vi "display_michelle_PKT_visjitter_stopadded_ContrastTitration.vi"() -> ()   [LabVIEW 2019]
uses:
  <vilib>/Analysis/Matrix/Datatypes/RealMatrix.ctl
  <vilib>/Utility/file.llb/Write Delimited Spreadsheet (DBL).vi
  <vilib>/Analysis/Matrix/NI_Matrix.lvlib
panel:
  out "lambda":dbl
  out "maxITI":dbl
  out "minITI":dbl
  out "goEXP":dbl
  out "Array temp3":T1
  out "OTDisp":dbl
  out "Performance":dbl
  out "CurrentContrast":dbl
  out "OTRew":dbl
  out "TrialGroup":dbl format="%#_13g"
  out "DisplayCount":dbl
  out "TimeOutCounter":i32
  out "ElapsedTime_M":dbl
  out "IMG_Contrast":dbl
  out "CurrentTrial":u32=1
  out "Jitter":dbl
  out "BaseITI":dbl
  out "VisStimDuration":dbl
  in  "Stop":bool
  out "Num trials":u32=204
  out "ISI Time":dbl
  out "Stim TS":dbl
  out "Output":dbl[][](array[numeric])
  out "Output frame":T1
  out "Array temp1":T1
  out "Elapsed Time":dbl
  out "Display":bool=TRUE
  out "Trial":u32=1
  out "reward":dbl[](array[numeric])
  out "stim_id":dbl[](array[numeric])
  out "stim_loaded":dbl
  out "Timings":dbl[](array[numeric])
  out "Stimuli Loaded?":bool
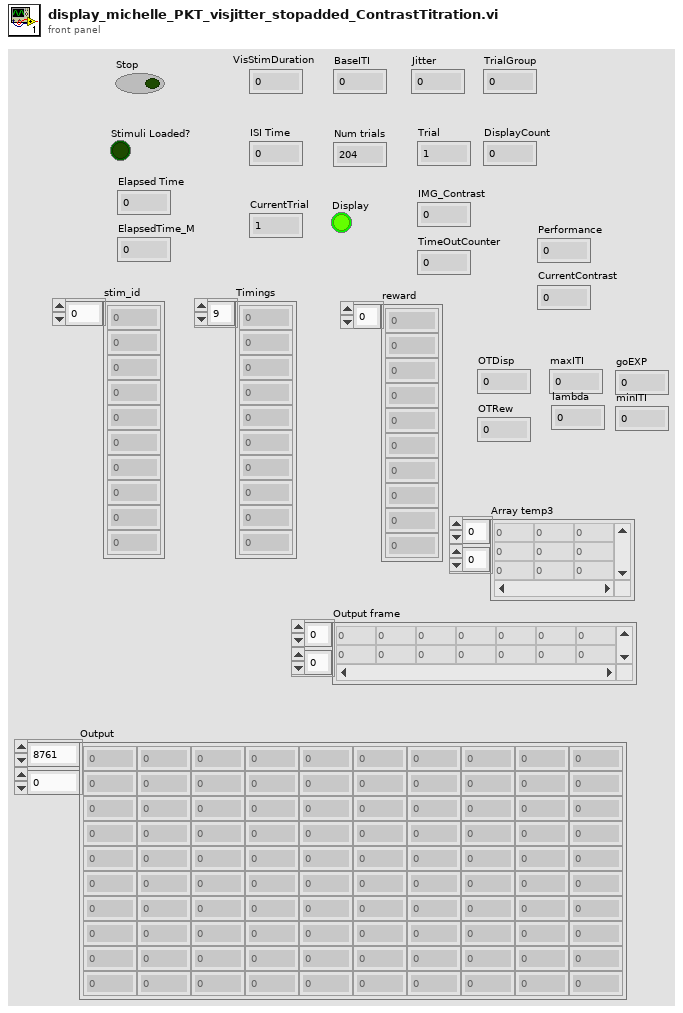
[diagram p1: front panel]
types:
  T1 = typedef "NI_Matrix.lvlib/RealMatrix.ctl" = dbl[][]
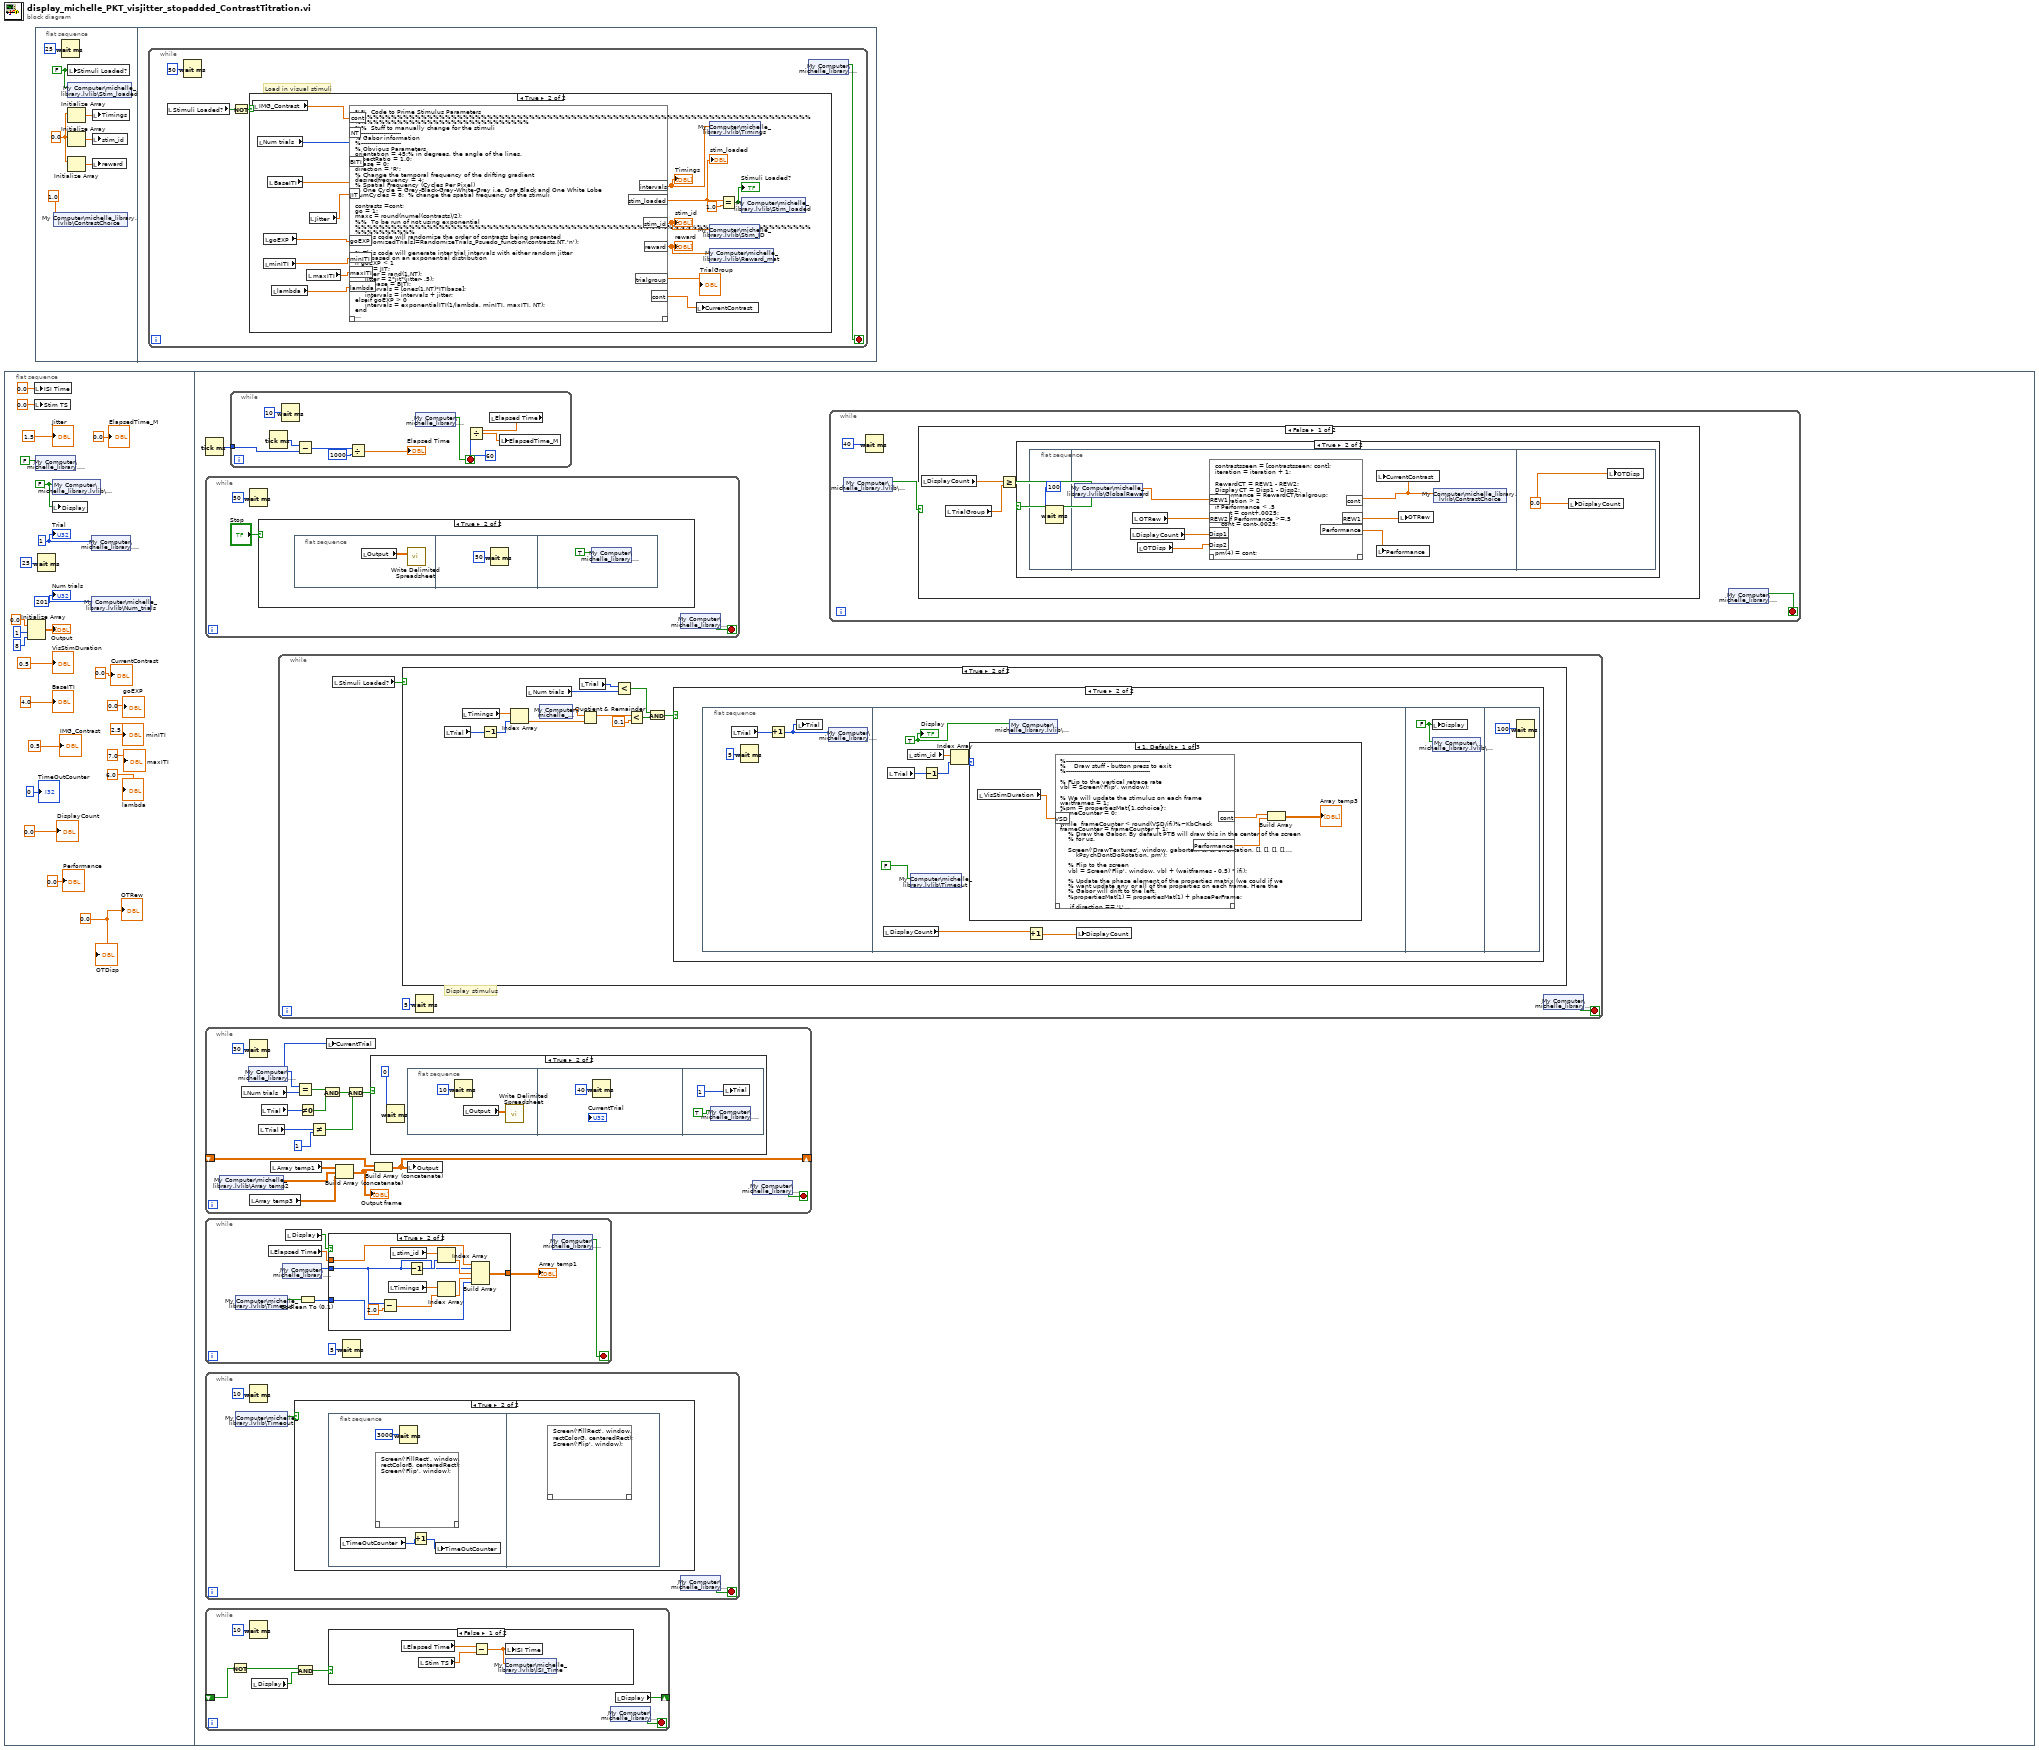
[diagram p0: block diagram]
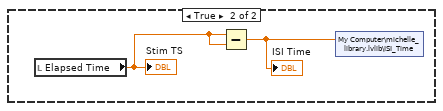
[diagram p7: hidden frame]
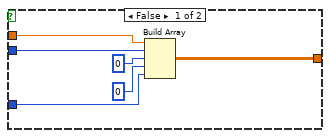
[diagram p8: hidden frame]
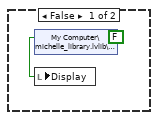
[diagram p11: hidden frame]
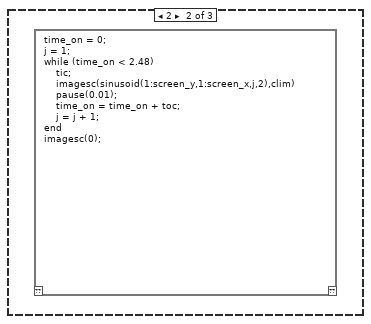
[diagram p12: hidden frame]
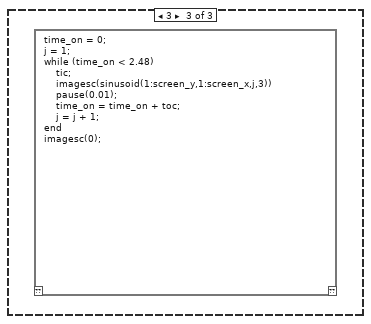
[diagram p13: hidden frame]
diagram:
  n1 = flat-sequence {
    frame #0 {
      w7 = 0.0
      w17 = u32 201
      w23 = FALSE ("Display")
      w25 = u32 1 ("Trial")
      n2 = Initialize Array(0.0 ("element"), 1 ("dimension size"), 8 ("dimension size")) -> (→"Output":dbl[][])
      n3 = local write "ISI Time"(0.0 ("ISI Time")) -> ()
      n4 = local write "Stim TS"(0.0 ("Stim TS")) -> ()
      n5 = shared-variable "My Computer\\michelle_library.lvlib\\Stop"(FALSE ("Stop")) -> ()  [unwired: 1 in, 1 out]
      n6 = Wait (ms)(milliseconds to wait=u32 25) -> ()  [unwired: 1 out]
      n7 = shared-variable "My Computer\\michelle_library.lvlib\\Display"(w23) -> ()  [unwired: 1 in, 1 out]
      n8 = local write "Display"(w23) -> ()
      n9 = shared-variable "My Computer\\michelle_library.lvlib\\Trial"(w25) -> ()  [unwired: 1 in, 1 out]
      n10 = shared-variable "My Computer\\michelle_library.lvlib\\Num_trials"(w17) -> ()  [unwired: 1 in, 1 out]
      "Trial" <- w25
      "Num trials" <- w17
      "VisStimDuration" <- 0.5
      "BaseITI" <- 4.0
      "Jitter" <- 1.5
      "IMG_Contrast" <- 0.5
      "ElapsedTime_M" <- 0.0
      "TimeOutCounter" <- 0
      "DisplayCount" <- 0.0
      "OTRew" <- w7
      "CurrentContrast" <- 0.0
      "Performance" <- 0.0
      "OTDisp" <- w7
      "goEXP" <- 0.0
      "minITI" <- 2.5
      "maxITI" <- 7.0
      "lambda" <- 6.0
    }
    frame #1 {
      n11 = Tick Count (ms)() -> (millisecond timer value=w26:u32)
      n12 = while {
        stop <- w44 stop-if-true
        n13 = Wait (ms)(milliseconds to wait=50) -> ()  [unwired: 1 out]
        n14 = case shown="True" "Stop" {
          frame False {
          }
          frame True {
            n15 = flat-sequence {
              frame #0 {
                n16 = local read "Output"() -> (w45:dbl[][])
                n17 = call-poly <vilib>:"Write Delimited Spreadsheet.vi"("2D data"=w45) -> ()  [unwired: 13 in, 2 out]
              }
              frame #1 {
                n18 = Wait (ms)(milliseconds to wait=50) -> ()  [unwired: 1 out]
              }
              frame #2 {
                n19 = shared-variable "My Computer\\michelle_library.lvlib\\Stop"(TRUE) -> ()  [unwired: 1 in, 1 out]
              }
            }
          }
        }
        n20 = shared-variable "My Computer\\michelle_library.lvlib\\Stop"() -> (w44:bool)  [unwired: 1 in, 1 out]
      }
      n21 = while {
        shift-right: [w115] -> _
        shift-left: _ -> [w116]
        stop <- w118 stop-if-true
        n22 = shared-variable "My Computer\\michelle_library.lvlib\\Array temp2"() -> (w113:dbl[][])  [unwired: 1 in, 1 out]
        n23 = local read "Num trials"() -> (w111:u32)
        n24 = shared-variable "My Computer\\michelle_library.lvlib\\Trial"() -> (w102:u32)  [unwired: 1 in, 1 out]
        n25 = Wait (ms)(milliseconds to wait=u32 30) -> ()  [unwired: 1 out]
        n26 = local read "Array temp3"() -> (w101:T1)
        n27 = local read "Trial"() -> (w108:u32)
        n28 = local read "Trial"() -> (w109:u32)
        n29 = local read "Array temp1"() -> (w114:T1)
        n30 = Equal?(x=w102, y=w111) -> (x = y?=w110:bool)
        n31 = Not Equal To 0?(x=w109) -> (x != 0?=w105:bool)
        n32 = Not Equal?(x=w108, y=1) -> (x != y?=w107:bool)
        n33 = And(x=w110, y=w105) -> (x .and. y?=w103:bool)
        n34 = local write "CurrentTrial"(w102) -> ()
        n35 = Build Array (concatenate)(w114, w113, w101) -> (w112:T1)
        "Output frame" <- w112
        n36 = And(x=w103, y=w107) -> (x .and. y?=w104:bool)
        n37 = case shown="True" w104 {
          frame False {
          }
          frame True {
            n38 = Wait (ms)(milliseconds to wait=0) -> ()  [unwired: 1 out]
            n39 = flat-sequence {
              frame #0 {
                n40 = Wait (ms)(milliseconds to wait=u32 10) -> ()  [unwired: 1 out]
                n41 = local read "Output"() -> (w121:dbl[][])
                n42 = call-poly <vilib>:"Write Delimited Spreadsheet.vi"("2D data"=w121) -> ()  [unwired: 13 in, 2 out]
              }
              frame #1 {
                n43 = Wait (ms)(milliseconds to wait=u32 40) -> ()  [unwired: 1 out]
              }
              frame #2 {
                n44 = shared-variable "My Computer\\michelle_library.lvlib\\Stop"(TRUE) -> ()  [unwired: 1 in, 1 out]
                n45 = local write "Trial"(1) -> ()
              }
            }
          }
        }
        n46 = Build Array (concatenate) ("Build Matrix")(w116, w112) -> (w115:T1)
        n47 = local write "Output"(w115) -> ()
        n48 = shared-variable "My Computer\\michelle_library.lvlib\\Stop"() -> (w118:bool)  [unwired: 1 in, 1 out]
      }
      n49 = while {
        stop <- w68 stop-if-true
        n50 = shared-variable "My Computer\\michelle_library.lvlib\\Timeout"() -> (w66:bool)  [unwired: 1 in, 1 out]
        n51 = local read "Elapsed Time"() -> (w72:dbl)
        n52 = shared-variable "My Computer\\michelle_library.lvlib\\Trial"() -> (w70:u32)  [unwired: 1 in, 1 out]
        n53 = local read "Display"() -> (w69:bool)
        n54 = Boolean To (0,1)(Boolean=w66) -> (0, 1=w67:i16)
        n55 = case shown="True" w69 {
          tunnel: w70 -> [w78 w81]
          tunnel: w72 -> [w79 w88]
          tunnel: [w77 w89] -> w71
          tunnel: w67 -> [w74 w83]
          frame False {
            n56 = Build Array(w79, w78, u32 0 ("milliseconds to wait"), 0, w74) -> (w77:T1)
          }
          frame True {
            n57 = Subtract(x=w81, y=2.0) -> (x-y=w80:dbl)
            n58 = local read "Timings"() -> (w86:dbl[])
            n59 = local read "stim_id"() -> (w90:dbl[])
            n60 = Decrement(x=w81) -> (x-1=w85:u32)
            n61 = Index Array(array=w90, index=w85) -> (element=w87:dbl)
            n62 = Index Array(array=w86, index=w80) -> (element=w84:dbl)
            n63 = Build Array(w88, w81, w87, w84, w83) -> (w89:T1)
          }
        }
        "Array temp1" <- w71
        n64 = Wait (ms)(milliseconds to wait=u32 5) -> ()  [unwired: 1 out]
        n65 = shared-variable "My Computer\\michelle_library.lvlib\\Stop"() -> (w68:bool)  [unwired: 1 in, 1 out]
      }
      n66 = while {
        stop <- w50 stop-if-true
        n67 = shared-variable "My Computer\\michelle_library.lvlib\\Timeout"() -> (w48:bool)  [unwired: 1 in, 1 out]
        n68 = Wait (ms)(milliseconds to wait=u32 10) -> ()  [unwired: 1 out]
        n69 = case shown="True" w48 {
          frame False {
          }
          frame True {
            n70 = flat-sequence {
              frame #0 {
                n71 = local read "TimeOutCounter"() -> (w52:i32)
                n72 = script code="Screen('FillRect', window, rectColorB, centeredRect);\nScreen('Flip', window);"() -> ()  [unwired: 1 in, 1 out]
                n73 = Wait (ms)(milliseconds to wait=u32 3000) -> ()  [unwired: 1 out]
                n74 = Increment(x=w52) -> (x+1=w51:i32)
                n75 = local write "TimeOutCounter"(w51) -> ()
              }
              frame #1 {
                n76 = script code="Screen('FillRect', window, rectColorG, centeredRect);\nScreen('Flip', window);"() -> ()  [unwired: 1 in, 1 out]
              }
            }
          }
        }
        n77 = shared-variable "My Computer\\michelle_library.lvlib\\Stop"() -> (w50:bool)  [unwired: 1 in, 1 out]
      }
      n78 = while {
        shift-right: [w58] -> _
        shift-left: _ -> [w57]
        stop <- w60 stop-if-true
        n79 = Not(x=w57) -> (.not. x?=w56:bool)
        n80 = Wait (ms)(milliseconds to wait=u32 10) -> ()  [unwired: 1 out]
        n81 = local read "Display"() -> (w55:bool)
        n82 = And(x=w56, y=w55) -> (x .and. y?=w54:bool)
        n83 = case shown="False" w54 {
          frame False {
            n84 = local read "Elapsed Time"() -> (w61:dbl)
            n85 = local read "Stim TS"() -> (w63:dbl)
            n86 = Subtract(x=w61, y=w63) -> (x-y=w62:dbl)
            n87 = local write "ISI Time"(w62) -> ()
            n88 = shared-variable "My Computer\\michelle_library.lvlib\\ISI_Time"(w62) -> ()  [unwired: 1 in, 1 out]
          }
          frame True {
            n89 = local read "Elapsed Time"() -> (w64:dbl)
            "Stim TS" <- w64
            n90 = Subtract(x=w64, y=w64) -> (x-y=w65:dbl)
            "ISI Time" <- w65
            n91 = shared-variable "My Computer\\michelle_library.lvlib\\ISI_Time"(w65) -> ()  [unwired: 1 in, 1 out]
          }
        }
        n92 = shared-variable "My Computer\\michelle_library.lvlib\\Stop"() -> (w60:bool)  [unwired: 1 in, 1 out]
        n93 = local read "Display"() -> (w58:bool)
      }
      n94 = while {
        tunnel: w26 -> [w97]
        stop <- w94 stop-if-true
        n95 = Tick Count (ms)() -> (millisecond timer value=w98:u32)
        n96 = Wait (ms)(milliseconds to wait=u32 10) -> ()  [unwired: 1 out]
        n97 = Subtract(x=w98, y=w97) -> (x-y=w95:u32)
        n98 = Divide(x=w95, y=u32 1000) -> (x/y=→"Elapsed Time":dbl)
        n99 = shared-variable "My Computer\\michelle_library.lvlib\\Stop"() -> (w94:bool)  [unwired: 1 in, 1 out]
        n100 = local read "Elapsed Time"() -> (w91:dbl)
        n101 = Divide(x=w91, y=60) -> (x/y=w93:dbl)
        n102 = local write "ElapsedTime_M"(w93) -> ()
      }
      n103 = while {
        stop <- w126 stop-if-true
        # "Display stimulus"
        n104 = local read "Stimuli Loaded?"() -> (w125:bool)
        n105 = case shown="True" w125 {
          frame False {
          }
          frame True {
            n106 = local read "Trial"() -> (w128:u32)
            n107 = local read "Timings"() -> (w137:dbl[])
            n108 = Decrement(x=w128) -> (x-1=w129:u32)
            n109 = Index Array(array=w137, index=w129) -> (element=w136:dbl)
            n110 = local read "Num trials"() -> (w132:u32)
            n111 = shared-variable "My Computer\\michelle_library.lvlib\\ISI"() -> (w131:dbl)  [unwired: 1 in, 1 out]
            n112 = local read "Trial"() -> (w135:u32)
            n113 = Quotient & Remainder(x=w131, y=w136) -> (x-y*floor(x/y)=w139:dbl)  [unwired: 1 out]
            n114 = Less?(x=w135, y=w132) -> (x < y?=w134:bool)
            n115 = Less?(x=w139, y=0.1) -> (x < y?=w133:bool)
            n116 = And(x=w134, y=w133) -> (x .and. y?=w130:bool)
            n117 = case shown="True" w130 {
              frame False {
                w140 = FALSE ("Display")
                n118 = shared-variable "My Computer\\michelle_library.lvlib\\Display"(w140) -> ()  [unwired: 1 in, 1 out]
                n119 = local write "Display"(w140) -> ()
              }
              frame True {
                n120 = flat-sequence {
                  frame #0 {
                    n121 = local read "Trial"() -> (w143:u32)
                    n122 = Wait (ms)(milliseconds to wait=u32 5) -> ()  [unwired: 1 out]
                    n123 = Increment(x=w143) -> (x+1=w142:u32)
                    n124 = local write "Trial"(w142) -> ()
                    n125 = shared-variable "My Computer\\michelle_library.lvlib\\Trial"(w142) -> ()  [unwired: 1 in, 1 out]
                  }
                  frame #1 {
                    w150 = TRUE ("Boolean")
                    n126 = local read "DisplayCount"() -> (w145:dbl)
                    n127 = local read "Trial"() -> (w148:u32)
                    n128 = local read "stim_id"() -> (w151:dbl[])
                    n129 = shared-variable "My Computer\\michelle_library.lvlib\\Timeout"(FALSE) -> ()  [unwired: 1 in, 1 out]
                    n130 = Decrement(x=w148) -> (x-1=w147:u32)
                    n131 = Index Array(array=w151, index=w147) -> (element=w149:dbl)
                    n132 = case shown="1, Default" w149 {
                      frame 1, Default {
                        n133 = local read "VisStimDuration"() -> (w155:dbl)
                        n134 = script code="%------------------------------------------\n%    Draw stuff - button press to exit\n%------------------------------------------\n\n% FLip to the vertical retrace rate\nvbl = Screen('Flip', window);\n\n% We will update the stimulus on each frame\nwaitframes = 1;\n%pm = propertiesMat{1,cchoice};\nframeCounter = 0;\ntic\nwhile  frameCounter < round(VSD/ifi)%~KbCheck\nframeCounter = frameCounter + 1;\n    % Draw the Gabor. By default PTB will draw this in the center of the screen\n    % for us.\n   \n    Screen('DrawTextures', window, gabortex, [], [], orientation, [], [], [], [],...\n        kPsychDontDoRotation, pm');\n\n    % Flip to the screen\n    vbl = Screen('Flip', window, vbl + (waitframes - 0.5) * ifi);\n\n    % Update the phase element of the properties matrix (we could if we\n    % want update any or all of the properties on each frame. Here the\n    % Gabor will drift to the left.\n    %propertiesMat(1) = propertiesMat(1) + phasePerFrame;\n \n     if direction == 'L'\n          pm(1) = pm(1) + phasePerFrame;\n     elseif direction =='R'\n          pm(1) = pm(1) - phasePerFrame;\n     end\n\nend\nTime(N) = toc;\nvbl = Screen('Flip', window);\npm(1) = 0;"("VSD"=w155) -> ("cont"=w154:dbl, "Performance"=w152:dbl)  [unwired: 1 in, 1 out]
                        n135 = Build Array(w154, w152) -> (→"Array temp3":T1)
                      }
                      frame 2 {
                        n136 = script code="time_on = 0;\nj = 1;\nwhile (time_on < 2.48)\n    tic;\n    imagesc(sinusoid(1:screen_y,1:screen_x,j,2),clim)\n    pause(0.01);\n    time_on = time_on + toc;\n    j = j + 1;\nend\nimagesc(0);"() -> ()  [unwired: 1 in, 1 out]
                      }
                      frame 3 {
                        n137 = script code="time_on = 0;\nj = 1;\nwhile (time_on < 2.48)\n    tic;\n    imagesc(sinusoid(1:screen_y,1:screen_x,j,3))\n    pause(0.01);\n    time_on = time_on + toc;\n    j = j + 1;\nend\nimagesc(0);"() -> ()  [unwired: 1 in, 1 out]
                      }
                    }
                    n138 = shared-variable "My Computer\\michelle_library.lvlib\\Display"(w150) -> ()  [unwired: 1 in, 1 out]
                    n139 = Increment(x=w145) -> (x+1=w144:dbl)
                    n140 = local write "DisplayCount"(w144) -> ()
                    "Display" <- w150
                  }
                  frame #2 {
                    w156 = FALSE ("Display")
                    n141 = local write "Display"(w156) -> ()
                    n142 = shared-variable "My Computer\\michelle_library.lvlib\\Display"(w156) -> ()  [unwired: 1 in, 1 out]
                  }
                  frame #3 {
                    n143 = Wait (ms)(milliseconds to wait=u32 100) -> ()  [unwired: 1 out]
                  }
                }
              }
            }
          }
        }
        n144 = Wait (ms)(milliseconds to wait=u32 5) -> ()  [unwired: 1 out]
        n145 = shared-variable "My Computer\\michelle_library.lvlib\\Stop"() -> (w126:bool)  [unwired: 1 in, 1 out]
      }
      n146 = while {
        stop <- w29 stop-if-true
        n147 = shared-variable "My Computer\\michelle_library.lvlib\\Display"() -> (w28:bool)  [unwired: 1 in, 1 out]
        n148 = Wait (ms)(milliseconds to wait=40) -> ()  [unwired: 1 out]
        n149 = case shown="False" w28 {
          frame False {
            n150 = local read "DisplayCount"() -> (w31:dbl)
            n151 = local read "TrialGroup"() -> (w32:dbl)
            n152 = Greater Or Equal?(x=w31, y=w32) -> (x >= y?=w30:bool)
            n153 = case shown="True" w30 {
              frame False {
              }
              frame True {
                n154 = flat-sequence {
                  frame #0 {
                    n155 = Wait (ms)(milliseconds to wait=100) -> ()  [unwired: 1 out]
                  }
                  frame #1 {
                    n156 = shared-variable "My Computer\\michelle_library.lvlib\\GlobalReward"() -> (w40:dbl)  [unwired: 1 in, 1 out]
                    n157 = local read "DisplayCount"() -> (w37:dbl)
                    n158 = local read "OTRew"() -> (w39:dbl)
                    n159 = local read "OTDisp"() -> (w38:dbl)
                    n160 = script code="contrastsseen = [contrastsseen; cont];\niteration = iteration + 1;\n\nRewardCT = REW1 - REW2;\nDisplayCT = Disp1 - Disp2;\nPerformance = RewardCT/trialgroup;\nif iteration > 2\nif Performance < .5\n  cont = cont+.0025;\nelseif Performance >=.5\n   cont = cont-.0025;\nend\nend\n\n\npm(4) = cont;"("REW1"=w40, "REW2"=w39, "Disp1"=w37, "Disp2"=w38) -> ("cont"=w34:dbl, "Performance"=w35:dbl, "REW1"=w36:dbl)  [unwired: 1 in, 1 out]
                    n161 = local write "Performance"(w35) -> ()
                    n162 = local write "CurrentContrast"(w34) -> ()
                    n163 = local write "OTRew"(w36) -> ()
                    n164 = shared-variable "My Computer\\michelle_library.lvlib\\ContrastChoice"(w34) -> ()  [unwired: 1 in, 1 out]
                  }
                  frame #2 {
                    w41 = 0.0
                    n165 = local write "DisplayCount"(w41) -> ()
                    n166 = local write "OTDisp"(w41) -> ()
                  }
                }
              }
            }
          }
          frame True {
          }
        }
        n167 = shared-variable "My Computer\\michelle_library.lvlib\\Stop"() -> (w29:bool)  [unwired: 1 in, 1 out]
      }
    }
  }
  n168 = flat-sequence {
    frame #0 {
      w161 = 0.0 ("element")
      w159 = FALSE ("Stimuli Loaded?")
      n169 = shared-variable "My Computer\\michelle_library.lvlib\\ContrastChoice"(1.0) -> ()  [unwired: 1 in, 1 out]
      n170 = Wait (ms)(milliseconds to wait=u32 25) -> ()  [unwired: 1 out]
      n171 = local write "Stimuli Loaded?"(w159) -> ()
      n172 = shared-variable "My Computer\\michelle_library.lvlib\\Stim_loaded"(w159) -> ()  [unwired: 1 in, 1 out]
      n173 = Initialize Array(w161) -> (w163:dbl[])  [unwired: 1 in]
      n174 = Initialize Array(w161) -> (w162:dbl[])  [unwired: 1 in]
      n175 = Initialize Array(w161) -> (w160:dbl[])  [unwired: 1 in]
      n176 = local write "Timings"(w163) -> ()
      n177 = local write "stim_id"(w162) -> ()
      n178 = local write "reward"(w160) -> ()
    }
    frame #1 {
      n179 = while {
        stop <- w167 stop-if-true
        # "Load in visual stimuli"
        n180 = local read "Stimuli Loaded?"() -> (w166:bool)
        n181 = Wait (ms)(milliseconds to wait=u32 50) -> ()  [unwired: 1 out]
        n182 = Not(x=w166) -> (.not. x?=w165:bool)
        n183 = case shown="True" w165 {
          frame False {
          }
          frame True {
            n184 = local read "IMG_Contrast"() -> (w175:dbl)
            n185 = local read "Num trials"() -> (w178:u32)
            n186 = local read "goEXP"() -> (w169:dbl)
            n187 = local read "minITI"() -> (w170:dbl)
            n188 = local read "BaseITI"() -> (w177:dbl)
            n189 = local read "lambda"() -> (w171:dbl)
            n190 = local read "maxITI"() -> (w172:dbl)
            n191 = local read "Jitter"() -> (w176:dbl)
            n192 = script code="%%  Code to Prime Stimulus Parameters\n%%%%%%%%%%%%%%%%%%%%%%%%%%%%%%%%%%%%%%%%%%%%%%%%%%%%%%%%%%%%%%%%%%%%%%%%%%%%%%%%%%%%%%%%%%%%%%%%%%%%%%%%%\n%%  Stuff to manually change for the stimuli\n%--------------------\n% Gabor information\n%--------------------\n% Obvious Parameters\norientation = 45;% in degrees, the angle of the lines.\naspectRatio = 1.0;\nphase = 0;\ndirection = 'R';\n% Change the temporal frequency of the drifting gradient\ndesiredfrequency = 4;\n% Spatial Frequency (Cycles Per Pixel)\n% One Cycle = Grey-Black-Grey-White-Grey i.e. One Black and One White Lobe\nnumCycles = 8;  % change the spatial frequency of the stimuli\n\ncontrasts =cont;\ngo = 1;\nmaxc = round(numel(contrasts)/2);\n%%  To be run of not using exponential\n%%%%%%%%%%%%%%%%%%%%%%%%%%%%%%%%%%%%%%%%%%%%%%%%%%%%%%%%%%%%%%%%%%%%%%%%%%%%%%%%%%%%%%\n% This code will randomize the order of contrasts being presented\n[RandomizedTrials]=RandomizeTrials_Psuedo_function(contrasts,NT,'n');\n\n% This code will generate inter trial intervals with either random jitter\n% or based on an exponential distribution\nif goEXP < 1\n     jit = JIT;\n     jitter = rand(1,NT);\n     jitter = 2*jit*(jitter- .5);\n     ITIbase = BITI;\n     intervals = [ones(1,NT)*ITIbase];\n     intervals = intervals + jitter;\nelseif goEXP > 0\n     intervals = exponentialITI(1/lambda, minITI, maxITI, NT);\nend\n\n%%  Prep the stimulus presentation software\n%%%%%%%%%%%%%%%%%%%%%%%%%%%%%%%%%%%%%%%%%%%%%%%%%%%%%%%%%%%%%%%%%%%%%%%%%%%\nsca;\nclose all;\n% Setup PTB with some default values\nPsychDefaultSetup(2);\n% Set the screen number to the external secondary monitor if there is one connected\nscreenNumber = max(Screen('Screens'));\n\n% Define black, white and grey\nwhite = WhiteIndex(screenNumber);\nblack = BlackIndex(screenNumber);\ngrey = white / 2;\n\n% Open the screen & define it's dimensions\n[window, windowRect] = PsychImaging('OpenWindow', screenNumber, grey,...\n    [], 32, 2, [], [], kPsychNeedRetinaResolution);\n[screenXpixels, screenYpixels] = Screen('WindowSize', window);\n[xCenter, yCenter] = RectCenter(windowRect);\n\n% Get the vertical refresh rate of the monitor\nifi = Screen('GetFlipInterval', window);\n\n% Set maximum priority level\ntopPriorityLevel = MaxPriority(window);\nPriority(topPriorityLevel);\n\n\n% Build a procedural gabor texture (Note: to get a \"standard\" Gabor patch\n% we set a grey background offset, disable normalisation, and set a\n% pre-contrast multiplier of 0.5).\n% Dimension of the region where will draw the Gabor in pixels\ngaborDimPix = windowRect(3);\n% Sigma of Gaussian  (how much to fade around the edges)\nsigma = gaborDimPix / 0;  % change the 0 value to alter the fading\nphasePerFrame = desiredfrequency*360*ifi;\nfreq = numCycles / gaborDimPix;\n\nbackgroundOffset = [0.5 0.5 0.5 0.0];\ndisableNorm = 1;\npreContrastMultiplier = 0.5;\ngabortex = CreateProceduralGabor(window, gaborDimPix, gaborDimPix, [],...\n    backgroundOffset, disableNorm, preContrastMultiplier);\n\n% Randomise the phase of the Gabors and make a properties matrix.\nfor N = 1:numel(contrasts)\npropertiesMat{1,N} = [phase, freq, sigma, contrasts(N), aspectRatio, 0, 0, 0];\nend\n\niiii = 1;\ncchoice = RandomizedTrials(iiii);\ncont2 = contrasts(cchoice);\npm = propertiesMat{1,1};\n\n\n%%  Build up the rectangles for the pause and hold screen\nbaseRect = [0 0 screenXpixels screenYpixels];\ncenteredRect = CenterRectOnPointd(baseRect, xCenter, yCenter);\nrectColorB = [0 0 0];\nrectColorG = [128 128 128]/255;\n\n%%  Finalize the trial data and orders\nstim_id = [ones(1,NT)*1];\nreward = [ones(1,NT)*1];\nmeanITI = nanmean(intervals);\nrand_idx1 = randperm(NT);\nrand_idx2 = randperm(NT);\nintervals = intervals(rand_idx2);\nstim_id = stim_id(rand_idx2);\nreward = reward(rand_idx2);\n%%  All Done!\n%  indicate that the necessary preloading of data has been completed.\nstim_loaded = 1;" ("Script Node")("NT"=w178, "BITI"=w177, "JIT"=w176, "cont"=w175, "goEXP"=w169, "minITI"=w170, "maxITI"=w172, "lambda"=w171) -> ("stim_loaded"=w184:dbl, "intervals"=w179:dbl[], "stim_id"=w180:dbl[], "reward"=w182:dbl[], "trialgroup"=→"TrialGroup":dbl, "cont"=w173:dbl)  [unwired: 1 in, 1 out]
            "stim_loaded" <- w184
            "Timings" <- w179
            "stim_id" <- w180
            "reward" <- w182
            n193 = local write "CurrentContrast"(w173) -> ()
            n194 = shared-variable "My Computer\\michelle_library.lvlib\\Timings"(w179) -> ()  [unwired: 1 in, 1 out]
            n195 = shared-variable "My Computer\\michelle_library.lvlib\\Stim_ID"(w180) -> ()  [unwired: 1 in, 1 out]
            n196 = shared-variable "My Computer\\michelle_library.lvlib\\Reward_mat"(w182) -> ()  [unwired: 1 in, 1 out]
            n197 = Equal?(x=w184, y=1.0) -> (x = y?=w181:bool)
            "Stimuli Loaded?" <- w181
            n198 = shared-variable "My Computer\\michelle_library.lvlib\\Stim_loaded"(w181) -> ()  [unwired: 1 in, 1 out]
          }
        }
        n199 = shared-variable "My Computer\\michelle_library.lvlib\\Stop"() -> (w167:bool)  [unwired: 1 in, 1 out]
      }
    }
  }
